vi "FSM_main.vi"() -> ()   [LabVIEW 2016]
panel:
  out "Functions":bool[](array[boolean])
  out "Current state":string
  out "Current Time":string
  in  "Manual turn off":bool
  in  "Event manual panel":bool
  out "Bool of state":bool[](array[boolean])
  # "Finte State Machine"
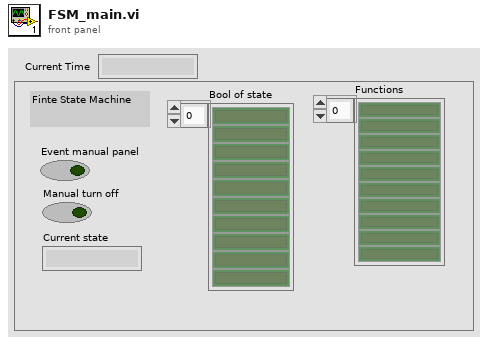
[diagram p1: front panel]
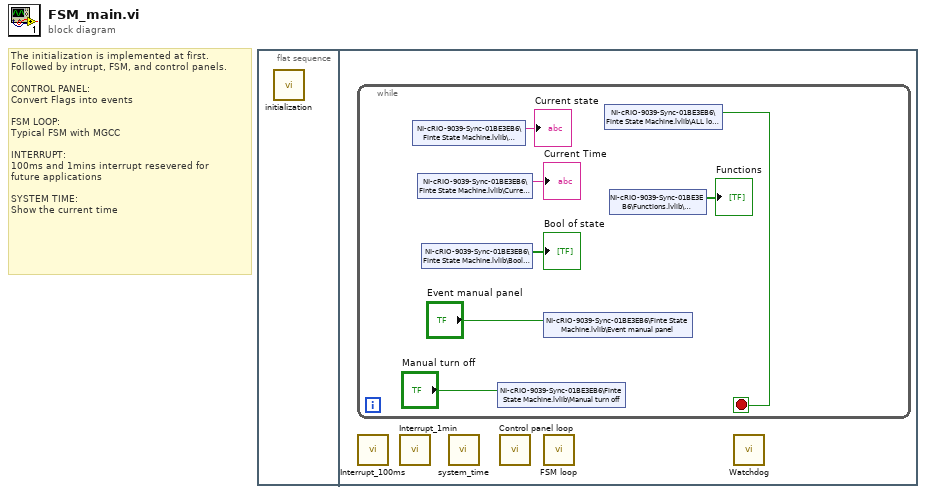
[diagram p0: block diagram]
diagram:
  # "The initialization is implemented at first.\nFollowed by intrupt, FSM, and control panels.\n\nCONTROL PANEL:\nConvert Flags into events\n\nFSM LOOP:\nTypical FSM with MGCC\n\nINTERRUPT:\n100ms and 1mins interrupt resevered for \nfuture applications\n\nSYSTEM TIME:\nShow the current time"
  n1 = flat-sequence {
    frame #0 {
      n2 = call "initialization.vi"() -> ()  [unwired: 12 in]
    }
    frame #1 {
      n3 = while {
        stop <- w6 stop-if-true
        n4 = shared-variable "NI-cRIO-9039-Sync-01BE3EB6\\Finte State Machine.lvlib\\Current state"() -> (→"Current state":string)  [unwired: 1 in, 1 out]
        n5 = shared-variable "NI-cRIO-9039-Sync-01BE3EB6\\Finte State Machine.lvlib\\Current Time"() -> (→"Current Time":string)  [unwired: 1 in, 1 out]
        n6 = shared-variable "NI-cRIO-9039-Sync-01BE3EB6\\Finte State Machine.lvlib\\Bool of state"() -> (→"Bool of state":bool[])  [unwired: 1 in, 1 out]
        n7 = shared-variable "NI-cRIO-9039-Sync-01BE3EB6\\Finte State Machine.lvlib\\Manual turn off"("Manual turn off") -> ()  [unwired: 1 in, 1 out]
        n8 = shared-variable "NI-cRIO-9039-Sync-01BE3EB6\\Finte State Machine.lvlib\\Event manual panel"("Event manual panel") -> ()  [unwired: 1 in, 1 out]
        n9 = shared-variable "NI-cRIO-9039-Sync-01BE3EB6\\Finte State Machine.lvlib\\ALL loop stop"() -> (w6:bool)  [unwired: 1 in, 1 out]
        n10 = shared-variable "NI-cRIO-9039-Sync-01BE3EB6\\Functions.lvlib\\Functions"() -> (→"Functions":bool[])  [unwired: 1 in, 1 out]
      }
      n11 = call "Interrupt_100ms.vi"() -> ()  [unwired: 11 in, 1 out]
      n12 = call "Interrupt_1min.vi"() -> ()  [unwired: 11 in, 1 out]
      n13 = call "system_time.vi"() -> ()  [unwired: 12 in]
      n14 = call "Control panel loop.vi"() -> ()  [unwired: 12 in]
      n15 = call "FSM loop.vi"() -> ()  [unwired: 6 in, 6 out]
      n16 = call "Watchdog.vi"() -> ()  [unwired: 12 in]
    }
  }
